vi "Close Session.vi"(8 "error in (no error)":errorcluster, 11 "MB TCP session":refnum<class "MB_Master_TCP.lvclass">) -> (0 "error out":errorcluster)   [LabVIEW 2012, in "MB Master.lvlib" / "MB_Master_TCP.lvclass"]
doc: "Close the Modbus session. This will release the mutex and close the TCP connection."
uses:
  MB_Master_TCP.lvclass
  MB_Master_TCP.lvclass/MB_Master_TCP.ctl
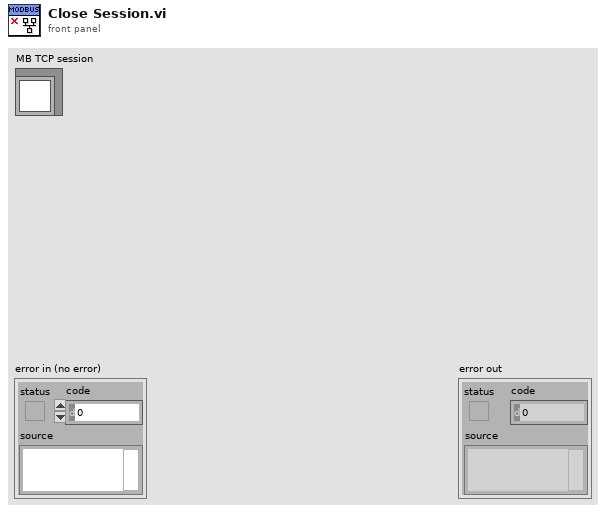
[diagram p1: front panel]
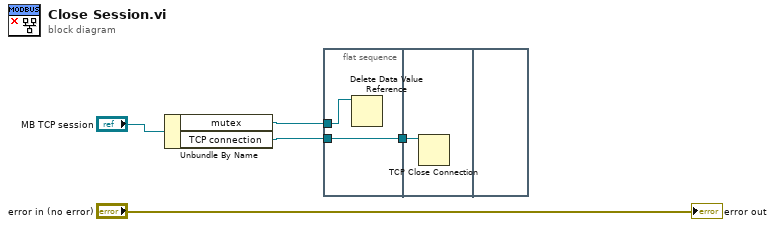
[diagram p0: block diagram]
diagram:
  n1 = Unbundle By Name("MB TCP session") -> ("mutex"=w1:refnum<data-value>, "TCP connection"=w4:refnum<k5>)
  n2 = flat-sequence {
    tunnel: w4 -> [w7]
    tunnel: [w7] -> w2
    tunnel: w1 -> [w6]
    tunnel: w2 -> [w8]
    frame #0 {
      n3 = Delete Data Value Reference(data value reference=w6) -> ()  [unwired: 1 in, 2 out]
    }
    frame #1 {
      n4 = TCP Close Connection(connection ID=w8) -> ()  [unwired: 2 in, 2 out]
    }
    frame #2 {
    }
  }
  "error out" <- "error in (no error)"
